vi "element_editor_close.vi"(11 "Close?":bool) -> ()   [LabVIEW 2019]
panel:
  # "*******************************************************************\nBiogas Plant Control\n\nAuthor: Paul Zügel\nGCSC-Frankfurt am Main 2020\n\n*******************************************************************"
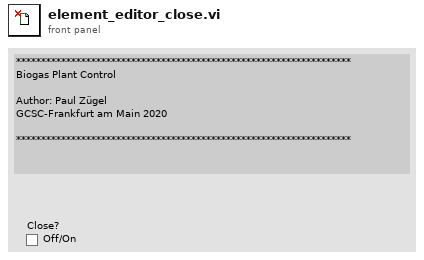
[diagram p1: front panel]
types:
  T1 = enum32{"Invalid", "Standard", "Closed", "Hidden", "Minimized", "Maximized"}
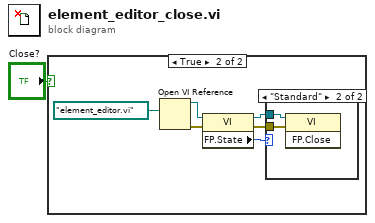
[diagram p0: block diagram]
diagram:
  n1 = case shown="True" "Close?" {
    frame False {
    }
    frame True {
      n2 = Open VI Reference(vi path=path "element_editor.vi") -> (vi reference=w3:refnum<vi>, error out=w2:errorcluster)  [unwired: 5 in]
      n3 = property class="VI"(reference=w3, error in=w2) -> (reference out=w5:refnum<vi>, error out=w4:errorcluster, "FP.State"=w6:T1)
      n4 = case shown="\"Standard\"" w6 {
        tunnel: w5 -> [_ w9]
        tunnel: w4 -> [_ w8]
        frame "Invalid", Default {
        }
        frame "Standard" {
          n5 = invoke class="VI" method="FP.Close"(reference=w9, error in=w8) -> ()  [unwired: 1 in, 3 out]
        }
      }
    }
  }
